vi "fgv_imu_config.vi"(7 "cmd":enum16{"read", "write"}(ring), 8 "error in":errorcluster, 11 "IMU cfg":T1={"Port"="COM10", "cmd"="", "rate"=115200}) -> (0 "error out":errorcluster, 3 "IMU cfg out":T1={"Port"="COM10", "cmd"="", "rate"=115200})   [LabVIEW 2019]
uses:
  Ctrl/imu-cfg.ctl
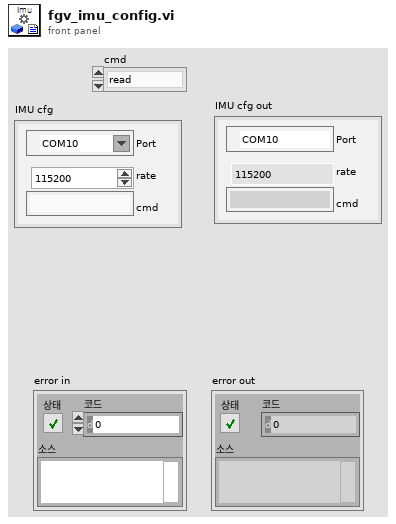
[diagram p1: front panel]
types:
  T1 = typedef "imu-cfg.ctl" = cluster{"Port":refnum<visa-resource-name>, "cmd":string, "rate":u32}
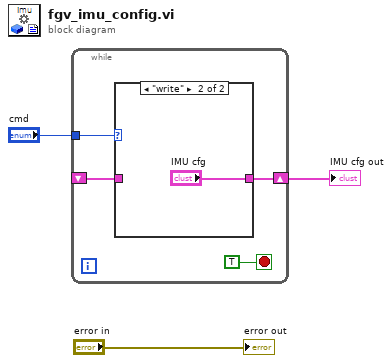
[diagram p0: block diagram]
diagram:
  n1 = while {
    tunnel: "cmd" -> [w6]
    shift-right: [w5] -> w1
    shift-left: _ -> [w4]
    stop <- TRUE stop-if-true
    n2 = case shown="\"write\"" w6 {
      tunnel: [w8 "IMU cfg"] -> w5
      tunnel: w4 -> [w8 _]
      frame "read", Default {
      }
      frame "write" {
      }
    }
  }
  "IMU cfg out" <- w1
  "error out" <- "error in"
